vi "Track Limelight Target (X Axis).vi"() -> (2 "Joystick X":dbl)   [LabVIEW 2019]
uses:
  <vilib>/Rock Robotics/Network Tables/NT Read Number.vi
  <vilib>/addons/control/pid/pid.llb/PID (DBL).vi
  <vilib>/addons/control/pid/NI_PID_pid.lvlib
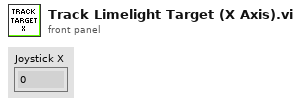
[diagram p1: front panel]
types:
  T1 = cluster{"proportional gain (Kc)":dbl, "integral time (Ti, min)":dbl, "derivative time (Td, min)":dbl}
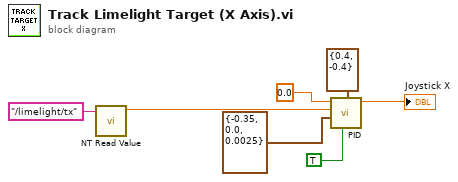
[diagram p0: block diagram]
diagram:
  n1 = call-poly <vilib>:"NT Read Value.vi"("Name"="/limelight/tx") -> ("Numeric"=w3:dbl)  [unwired: 9 in, 1 out]
  n2 = call-poly <vilib>:"PID.vi"("reinitialize? (F)"=TRUE, "output range"=cluster{"output high":dbl, "output low":dbl} {"output high"=0.4, "output low"=-0.4}, "PID gains"=T1 {"proportional gain (Kc)"=-0.35, "integral time (Ti, min)"=0.0, "derivative time (Td, min)"=0.0025}, "process variable"=w3, "setpoint"=0.0) -> ("output"=→"Joystick X":dbl)  [unwired: 5 in, 1 out]
